vi "PathDialog.vi"() -> (3 "Path 2out":path)   [LabVIEW 2016]
panel:
  in  "OK Button":bool
  in  "Path":path
  # "Select your PYBD volume"
  # "Click on the Browse button"
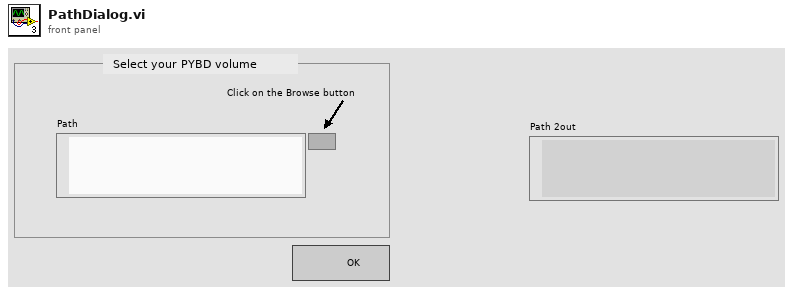
[diagram p1: front panel]
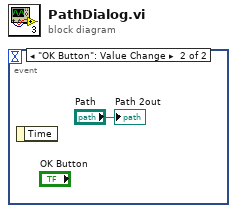
[diagram p0: block diagram]
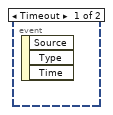
[diagram p2: hidden frame]
diagram:
  n1 = event shown="[1] \"OK Button\": Value Change" {
    selector: _ -> [_ _]
    dyn-events: _ -> [_ _]
    timeout: _ -> [_ _]
    event Timeout {
      n2 = event-data() -> ()  [unwired: 1 in, 3 out]
    }
    event "OK Button": Value Change {
      n3 = event-data() -> ()  [unwired: 1 in, 1 out]
      "Path 2out" <- "Path"
    }
  }
